vi "Data_formating.vi"(10 "String":string) -> (0 "Result string":string, 1 "Space not found?":bool, 2 "Response":string, 3 "Negative response?":bool)   [LabVIEW 2022 SP3]
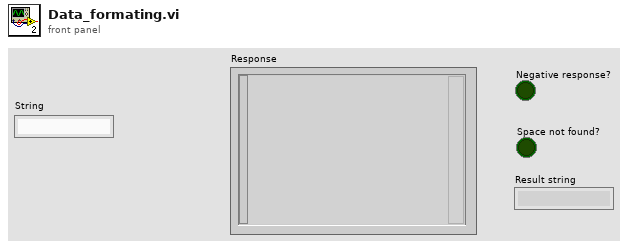
[diagram p1: front panel]
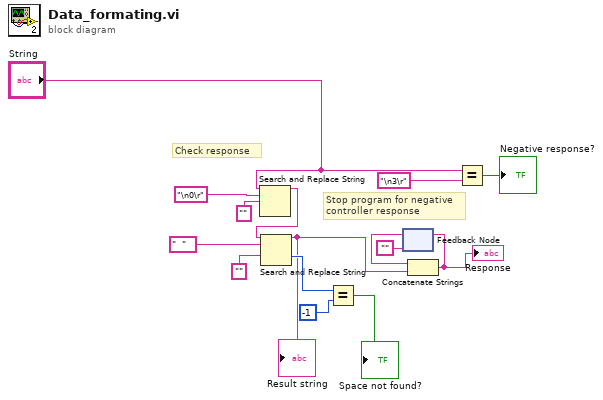
[diagram p0: block diagram]
diagram:
  # "Check response"
  # "Stop program for negative\ncontroller response"
  n1 = Search and Replace String(input string="String", search string="\n0\r" ("regular expression (\"\")"), replace string="" ("replace string (\"\")")) -> (result string=w10:string)  [unwired: 5 in, 3 out]
  n2 = Search and Replace String(input string=w10, search string="  " ("regular expression (\"\")"), replace string="" ("replace string (\"\")")) -> (result string=w5:string, offset past replacement=w9:i32)  [unwired: 5 in, 2 out]
  "Result string" <- w5
  n3 = Equal?(x=w9, y=-1) -> (x = y?=→"Space not found?":bool)
  n4 = feedback #1("") -> (w7:string)
  n5 = Concatenate Strings(w7, w5) -> (w8:string)
  "Response" <- w8
  n6 = feedback-in #1(w8) -> ()
  n7 = Equal?(x="String", y="\n3\r" ("regular expression (\"\")")) -> (x = y?=→"Negative response?":bool)
